vi "DAQ 2장 실습 1-1_Sampling Rate Example.vi"() -> ()   [LabVIEW 2020]
uses:
  <vilib>/DAQmx/write.llb/DAQmx Write (Analog 1D DBL 1Chan NSamp).vi
  <vilib>/DAQmx/read.llb/DAQmx Read (Analog Wfm 1Chan NSamp).vi
  <vilib>/DAQmx/create/channels.llb/DAQmx Create Channel (AO-Voltage-Basic).vi
  <vilib>/DAQmx/create/channels.llb/DAQmx Create Channel (AI-Voltage-Basic).vi
  <vilib>/DAQmx/configure/timing.llb/DAQmx Timing (Sample Clock).vi
  <vilib>/DAQmx/miscellaneous.llb/DAQmx Fill In Error Info.vi
  <vilib>/measure/maspectr.llb/FFT Power Spectrum for 1 Chan.vi
  <vilib>/measure/NI_MAPro.lvlib
  <vilib>/Analysis/NI_AALBase.lvlib
  <resource>/objmgr/daqmx.rc
panel:
  in  "DAQmx 디바이스 이름":tag="Dev1"
  in  "아날로그 출력 주파수(Hz)":dbl(knob)=50.0 min=10.0 max=500.0 scale=50.0..500.0
  in  "아날로그 입력 주파수 (Hz)":dbl(knob)=100.0 min=100.0 max=5000.0 scale=100.0..5000.0
  in  "정지":bool
  out "주파수 영역 데이터":cluster{"f0":dbl, "df":dbl, "magnitude":dbl[]}(graph)={"f0"=0.0, "df"=1.0, "magnitude"=[]}
  out "시간 영역 데이터":waveform(dbl)(graph)={"t0"=timestamp(3661848008.3173184 s since 1904-01-01), "dt"=0.01, "Y"=[], "attributes"=variant("NI_ChannelName"=variant(string "Dev2/ai0"), "NI_UnitDescription"=variant(string "Volts"))}
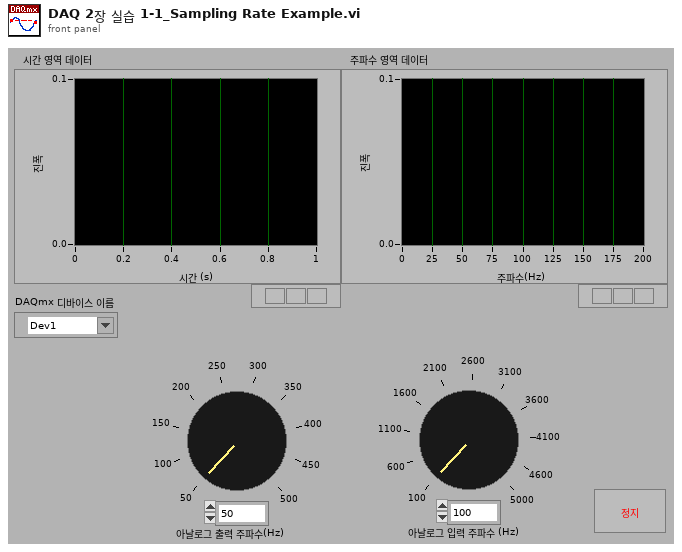
[diagram p1: front panel]
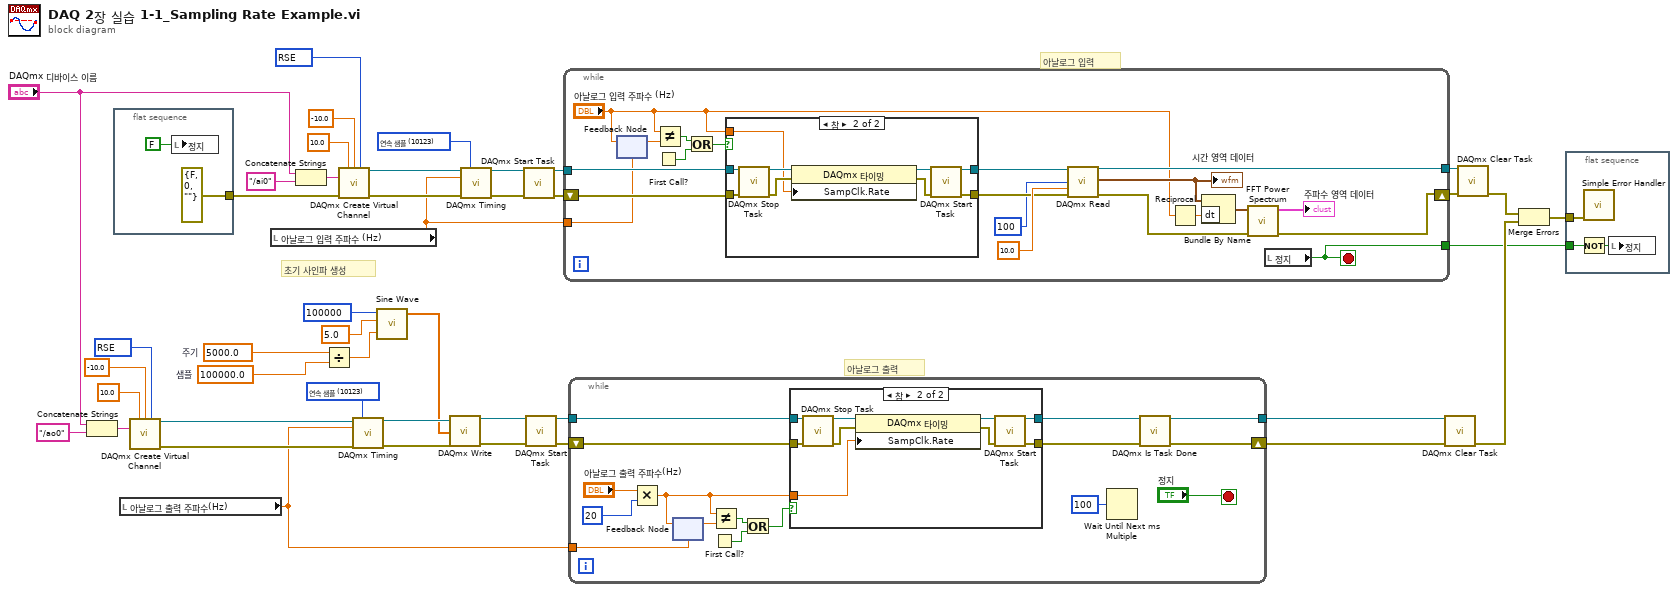
[diagram p0: block diagram]
diagram:
  w1 = 10083 items=["Default"=-1, "RSE"=10083, "Differential"=10106, "Pseudodifferential"=12529] ("output terminal configuration")
  w4 = 10083 items=["Default"=-1, "RSE"=10083, "NRSE"=10078, "Differential"=10106, "Pseudodifferential"=12529] ("input terminal configuration")
  w7 = 10123 items=["유한 샘플"=10178, "연속 샘플"=10123, "하드웨어 타이밍에 의한 단일 포인트"=12522] ("sample mode")
  w8 = 10123 items=["유한 샘플"=10178, "연속 샘플"=10123, "하드웨어 타이밍에 의한 단일 포인트"=12522] ("sample mode")
  w33 = 5000.0  # 주기
  w35 = 100000.0  # 샘플
  # "아날로그 출력"
  # "아날로그 입력"
  # "초기 사인파 생성"
  n1 = Concatenate Strings ("문자열 연결")("DAQmx 디바이스 이름", "/ao0" ("문자열")) -> (w12:string)
  n2 = flat-sequence {
    tunnel: [cluster{"상태":bool, "코드":i32, "소스":string} {"상태"=FALSE, "코드"=0, "소스"=""} ("에러 입력")] -> w17
    frame #0 {
      n3 = local write "정지"(FALSE ("정지")) -> ()
    }
  }
  n4 = local read "아날로그 출력 주파수(Hz)"() -> (w5:dbl)
  n5 = call-poly <vilib>:"DAQmx Create Virtual Channel.vi"("maximum value"=10.0, "minimum value"=-10.0, "output terminal configuration"=w1, "physical channels"=w12) -> ("task out"=w26:refnum<k21>, "error out"=w6:errorcluster)  [unwired: 10 in]
  n6 = local read "아날로그 입력 주파수 (Hz)"() -> (w10:dbl)
  n7 = Concatenate Strings ("문자열 연결")("DAQmx 디바이스 이름", "/ai0" ("문자열")) -> (w14:string)
  n8 = Divide ("나누기")(x=w33, y=w35) -> (x/y=w34:dbl)
  n9 = call-poly <vilib>:"DAQmx Create Virtual Channel.vi"("maximum value"=10.0 ("최대값"), "minimum value"=-10.0 ("최소값"), "input terminal configuration"=w4, "physical channels"=w14, "error in"=w17) -> ("task out"=w42:refnum<k21>, "error out"=w11:errorcluster)  [unwired: 9 in]
  n10 = call-poly <vilib>:"DAQmx Timing.vi"("task/channels in"=w26, "sample mode"=w7, "rate"=w5, "error in"=w6) -> ("task out"=w37:refnum<k21>, "error out"=w36:errorcluster)  [unwired: 10 in]
  n11 = call <vilib>:"Sine Wave.vi"("samples"=100000 ("샘플"), "amplitude"=5.0 ("진폭"), "frequency"=w34) -> ("sine wave"=w30:dbl[])  [unwired: 2 in, 2 out]
  n12 = call-poly <vilib>:"DAQmx Write.vi"("task/channels in"=w37, "data"=w30, "error in"=w36) -> ("task out"=w25:refnum<k21>, "error out"=w24:errorcluster)  [unwired: 10 in, 1 out]
  n13 = call-poly <vilib>:"DAQmx Timing.vi"("task/channels in"=w42, "sample mode"=w8, "rate"=w10, "error in"=w11) -> ("task out"=w27:refnum<k21>, "error out"=w41:errorcluster)  [unwired: 10 in]
  n14 = call <vilib>:"DAQmx Start Task.vi"("task/channels in"=w27, "error in"=w41) -> ("task out"=w40:refnum<k21>, "error out"=w39:errorcluster)  [unwired: 12 in]
  n15 = call <vilib>:"DAQmx Start Task.vi"("task/channels in"=w25, "error in"=w24) -> ("task out"=w29:refnum<k21>, "error out"=w28:errorcluster)  [unwired: 12 in]
  n16 = while {
    tunnel: w40 -> [w58]
    tunnel: [w65] -> w21
    tunnel: w10 -> [w50]
    tunnel: [w49] -> w9
    shift-right: [w64] -> w22
    shift-left: w39 -> [w55]
    stop <- w49 stop-if-true
    n17 = feedback-in #1("아날로그 입력 주파수 (Hz)") -> ()
    n18 = feedback #1(w50) -> (w54:dbl)
    n19 = First Call? ("첫번째 호출?")() -> (First Call?: T/F=w51:bool)
    n20 = Not Equal? ("같지 않음?")(x="아날로그 입력 주파수 (Hz)", y=w54) -> (x != y?=w53:bool)
    n21 = Or(x=w53, y=w51) -> (x .or. y?=w52:bool)
    n22 = case shown="참" w52 {
      tunnel: w58 -> [w68 w73]
      tunnel: w55 -> [w67 w72]
      tunnel: [w68 w71] -> w57
      tunnel: [w67 w70] -> w56
      tunnel: "아날로그 입력 주파수 (Hz)" -> [_ w69]
      frame False {
      }
      frame True {
        n23 = call <vilib>:"DAQmx Stop Task.vi"("task/channels in"=w73, "error in"=w72) -> ("task out"=w75:refnum<k21>, "error out"=w74:errorcluster)  [unwired: 12 in]
        n24 = property on="프로퍼티 노드" class="DAQmx 타이밍"(reference=w75, error in=w74, "SampClk.Rate"=w69) -> (reference out=w77:refnum<k21>, error out=w76:errorcluster)
        n25 = call <vilib>:"DAQmx Start Task.vi"("task/channels in"=w77, "error in"=w76) -> ("task out"=w71:refnum<k21>, "error out"=w70:errorcluster)  [unwired: 12 in]
      }
    }
    n26 = call-poly <vilib>:"DAQmx Read.vi"("task/channels in"=w57, "number of samples per channel"=100 ("채널당 샘플 개수"), "timeout"=10.0 ("타임아웃"), "error in"=w56) -> ("task out"=w65:refnum<k21>, "data"=w62:waveform(dbl), "error out"=w59:errorcluster)  [unwired: 9 in]
    "시간 영역 데이터" <- w62
    n27 = Reciprocal ("역수")(x="아날로그 입력 주파수 (Hz)") -> (1/x=w61:dbl)
    n28 = Bundle By Name ("웨이브폼 만들기")(cluster=w62, "dt"=w61) -> (w60:waveform(dbl))
    n29 = call-poly <vilib>:"FFT Power Spectrum.vi"("error in (no error)"=w59, "time signal"=w60) -> ("error out"=w64:errorcluster, "power spectrum"=→"주파수 영역 데이터":cluster{"f0":dbl, "df":dbl, "magnitude":dbl[]})  [unwired: 6 in, 2 out]
    n30 = local read "정지"() -> (w49:bool)
  }
  n31 = while {
    tunnel: w29 -> [w87]
    shift-right: [w90] -> w38
    shift-left: w28 -> [w86]
    tunnel: [w91] -> w23
    tunnel: w5 -> [w81]
    stop <- "정지" stop-if-true
    n32 = Multiply ("곱하기")(x="아날로그 출력 주파수(Hz)", y=20) -> (x*y=w79:dbl)
    n33 = feedback #2(w81) -> (w83:dbl)
    n34 = feedback-in #2(w79) -> ()
    n35 = First Call? ("첫번째 호출?")() -> (First Call?: T/F=w80:bool)
    n36 = Not Equal? ("같지 않음?")(x=w79, y=w83) -> (x != y?=w82:bool)
    n37 = Or(x=w82, y=w80) -> (x .or. y?=w78:bool)
    n38 = case shown="참" w78 {
      tunnel: w87 -> [w95 w100]
      tunnel: w86 -> [w94 w99]
      tunnel: [w95 w98] -> w85
      tunnel: [w94 w97] -> w84
      tunnel: w79 -> [_ w96]
      frame False {
      }
      frame True {
        n39 = call <vilib>:"DAQmx Stop Task.vi"("task/channels in"=w100, "error in"=w99) -> ("task out"=w102:refnum<k21>, "error out"=w101:errorcluster)  [unwired: 12 in]
        n40 = property on="프로퍼티 노드" class="DAQmx 타이밍"(reference=w102, error in=w101, "SampClk.Rate"=w96) -> (reference out=w104:refnum<k21>, error out=w103:errorcluster)
        n41 = call <vilib>:"DAQmx Start Task.vi"("task/channels in"=w104, "error in"=w103) -> ("task out"=w98:refnum<k21>, "error out"=w97:errorcluster)  [unwired: 12 in]
      }
    }
    n42 = Wait Until Next ms Multiple ("다음 ms 배수까지 기다림")(millisecond multiple=u32 100 ("밀리초 배수")) -> ()  [unwired: 1 out]
    n43 = call <vilib>:"DAQmx Is Task Done.vi"("task/channels in"=w85, "error in"=w84) -> ("task out"=w91:refnum<k21>, "error out"=w90:errorcluster)  [unwired: 11 in, 1 out]
  }
  n44 = call <vilib>:"DAQmx Clear Task.vi"("task in"=w23, "error in"=w38) -> ("error out"=w19:errorcluster)  [unwired: 13 in]
  n45 = call <vilib>:"DAQmx Clear Task.vi"("task in"=w21, "error in"=w22) -> ("error out"=w20:errorcluster)  [unwired: 13 in]
  n46 = Merge Errors ("에러 병합")(w20, w19) -> (w18:errorcluster)
  n47 = flat-sequence {
    tunnel: w18 -> [w107]
    tunnel: w9 -> [w105]
    frame #0 {
      n48 = Not(x=w105) -> (.not. x?=w106:bool)
      n49 = call <vilib>:"Simple Error Handler.vi"("error in (no error)"=w107) -> ()  [unwired: 4 in, 5 out]
      n50 = local write "정지"(w106) -> ()
    }
  }
